vi "Write CAN Frame.vi"(8 "error in (no error)":errorcluster, 10 "CAN Frame Array":T1(array[cluster]) {"payload" format="%.0x"; "identifier" format="%.0x"}, 11 "CAN Data in":refnum<class "CAN Data.lvclass">) -> (0 "error out":errorcluster, 3 "CAN Data out":refnum<class "CAN Data.lvclass">)   [LabVIEW 2021, in "BS120x Driver.lvlib" / "Data Classes.lvlib" / "CAN Data.lvclass"]
uses:
  CAN Data.lvclass
  CAN Data.lvclass/CAN Data.ctl
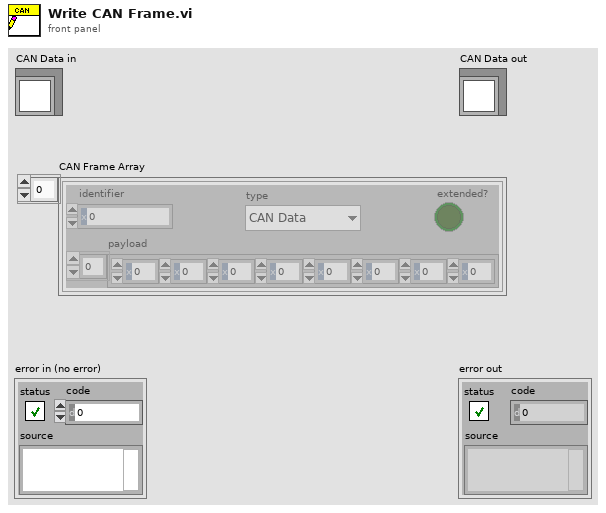
[diagram p1: front panel]
types:
  T1 = cluster{"identifier":u32, "extended?":bool, "type":enum8{"CAN Data", "CAN Remote"}, "payload":u8[]}[]
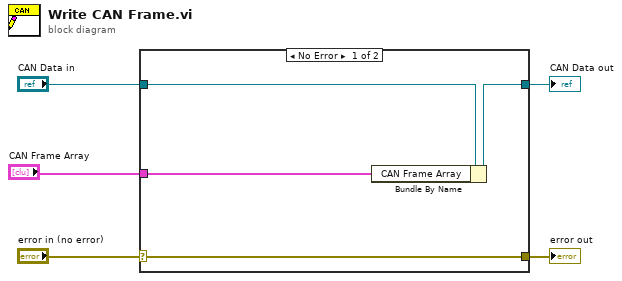
[diagram p0: block diagram]
diagram:
  n1 = case shown="No Error" "error in (no error)" {
    selector: "error in (no error)" -> [w9 w10]
    tunnel: [w9 w10] -> w4
    tunnel: [w7 w11] -> w2
    tunnel: "CAN Data in" -> [w8 w11]
    tunnel: "CAN Frame Array" -> [w6 _]
    frame No Error {
      n2 = Bundle By Name(cluster=w8, "CAN Frame Array"=w6) -> (w7:refnum<class "CAN Data.lvclass">)
    }
    frame Error {
    }
  }
  "error out" <- w4
  "CAN Data out" <- w2
